vi "Telnet Parse AIC Command.vi"(11 "AIC sequence":string) -> (0 "error":bool, 1 "command":string, 2 "after sequence":string, 3 "AIC result":string, 4 "option negotiation":bool, 5 "sub option negotiation":bool, 6 "option info":T1)   [LabVIEW 2014]
panel:
  out "Recved /FF/FE":bool
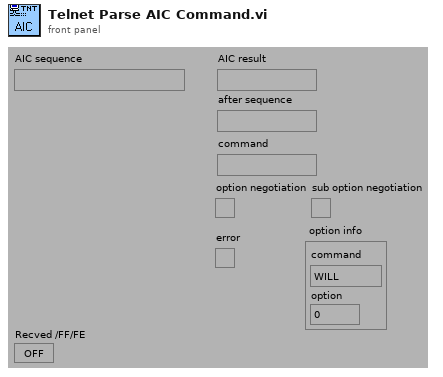
[diagram p1: front panel]
types:
  T1 = cluster{"command":enum16{"WILL", "WON'T", "DO", "DON'T"}, "option":u8}
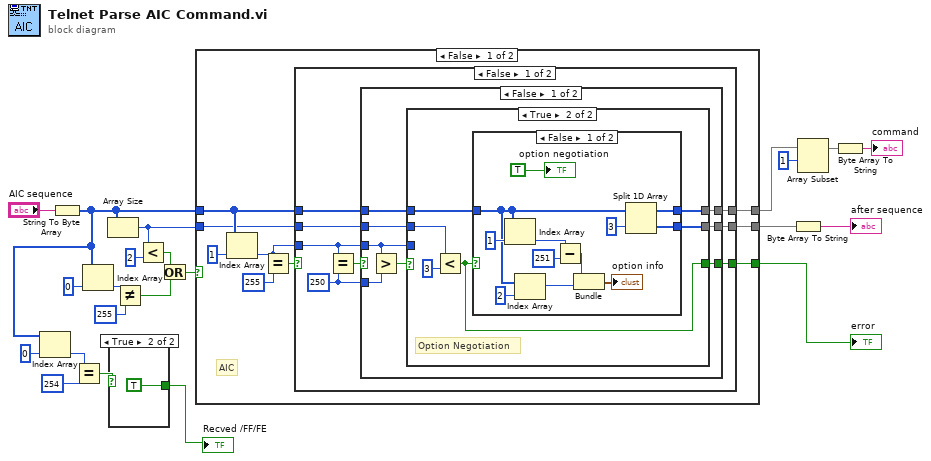
[diagram p0: block diagram]
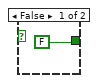
[diagram p2: hidden frame]
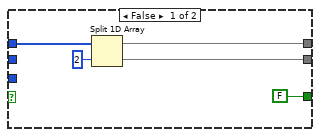
[diagram p3: hidden frame]
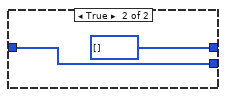
[diagram p4: hidden frame]
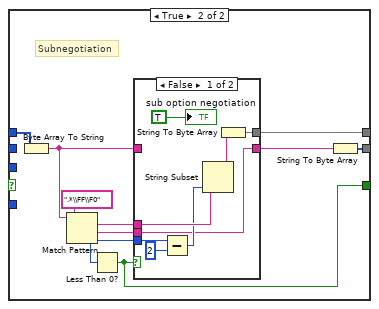
[diagram p5: hidden frame]
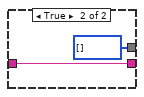
[diagram p6: hidden frame]
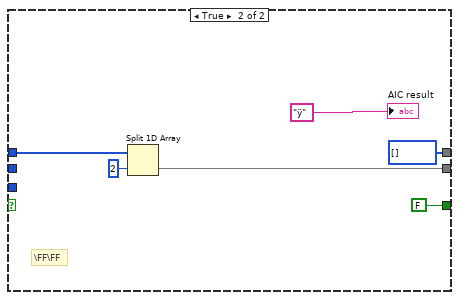
[diagram p7: hidden frame]
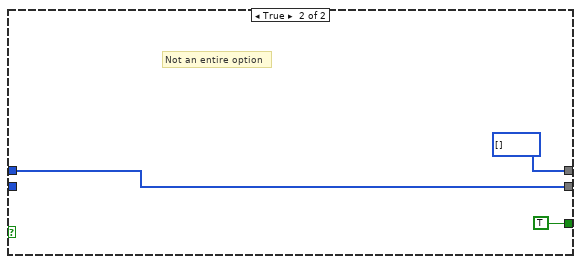
[diagram p8: hidden frame]
diagram:
  n1 = String To Byte Array(string="AIC sequence") -> (unsigned byte array=w5:u8[])
  n2 = Index Array(array=w5, index=0) -> (element=w4:u8)
  n3 = Equal?(x=w4, y=u8 254 ("x")) -> (x = y?=w2:bool)
  n4 = Index Array(array=w5, index=0) -> (element=w19:u8)
  n5 = Array Size(array=w5) -> (size(s)=w11:i32)
  n6 = case shown="True" w2 {
    tunnel: [FALSE TRUE] -> w1
    frame False {
    }
    frame True {
    }
  }
  "Recved /FF/FE" <- w1
  n7 = Not Equal?(x=w19, y=u8 255 ("x")) -> (x != y?=w18:bool)
  n8 = Less?(x=w11, y=2) -> (x < y?=w12:bool)
  n9 = Or(x=w12, y=w18) -> (x .or. y?=w13:bool)
  n10 = case shown="False" w13 {
    tunnel: w5 -> [w29 w102]
    tunnel: [w28 w102] -> w17
    tunnel: w11 -> [w27 _]
    tunnel: [w26 u8[] [] ("unsigned byte array")] -> w9
    tunnel: [w25 TRUE] -> w14
    frame False {
      # "AIC"
      n11 = Index Array(array=w29, index=1) -> (element=w31:u8)
      n12 = Equal?(x=w31, y=u8 255 ("x")) -> (x = y?=w30:bool)
      n13 = case shown="False" w30 {
        tunnel: w31 -> [w40 _]
        tunnel: w29 -> [w38 w100]
        tunnel: [w37 w98] -> w28
        tunnel: w27 -> [w36 _]
        tunnel: [w35 u8[] []] -> w26
        tunnel: [w34 FALSE] -> w25
        frame False {
          w41 = u8 250 ("x")
          n14 = Equal?(x=w40, y=w41) -> (x = y?=w39:bool)
          n15 = case shown="False" w39 {
            tunnel: w40 -> [w45 _]
            tunnel: w41 -> [w49 _]
            tunnel: w38 -> [w47 w84]
            tunnel: [w46 w82] -> w37
            tunnel: w36 -> [w44 _]
            tunnel: [w43 w76] -> w35
            tunnel: [w42 w75] -> w34
            frame False {
              n16 = Greater?(x=w45, y=w49) -> (0:w48:bool)
              n17 = case shown="True" w48 {
                tunnel: w47 -> [w54 w58]
                tunnel: [w52 w57] -> w46
                tunnel: w45 -> [_ _]
                tunnel: w44 -> [_ w59]
                tunnel: [w50 w56] -> w43
                tunnel: [FALSE w55] -> w42
                frame False {
                  n18 = Split 1D Array(array=w54, index=2) -> (first subarray=w50:u8[], second subarray=w52:u8[])
                }
                frame True {
                  # "Option Negotiation"
                  n19 = Less?(x=w59, y=3) -> (x < y?=w55:bool)
                  n20 = case shown="False" w55 {
                    tunnel: w58 -> [w62 w74]
                    tunnel: [w71 w74] -> w57
                    tunnel: [w70 u8[] []] -> w56
                    frame False {
                      n21 = Index Array(array=w62, index=1) -> (element=w67:u8)
                      n22 = Index Array(array=w62, index=2) -> (element=w61:u8)
                      n23 = Subtract(x=w67, y=u8 251) -> (x-y=w64:u8)
                      n24 = Bundle(w64, w61) -> (→"option info":cluster{u8, u8})  [unwired: 1 in]
                      n25 = Split 1D Array(array=w62, index=3) -> (first subarray=w70:u8[], second subarray=w71:u8[])
                      "option negotiation" <- TRUE ("option negotiation")
                    }
                    frame True {
                    }
                  }
                }
              }
            }
            frame True {
              # "Subnegotiation"
              n26 = Byte Array To String(unsigned byte array=w84) -> (string=w78:string)
              n27 = Match Pattern(string=w78, regular expression=".*\\FF\\F0") -> (match substring=w80:string, after substring=w77:string, offset past match=w81:i32)  [unwired: 1 in, 1 out]
              n28 = Less Than 0?(x=w81) -> (x < 0?=w75:bool)
              n29 = case shown="False" w75 {
                tunnel: w80 -> [w92 _]
                tunnel: w81 -> [w91 _]
                tunnel: [w88 w94] -> w79
                tunnel: w78 -> [_ w94]
                tunnel: w77 -> [w88 _]
                tunnel: [w86 u8[] [] ("unsigned byte array")] -> w76
                frame False {
                  n30 = Subtract(x=w91, y=2) -> (x-y=w89:i32)
                  n31 = String Subset(string=w92, length (rest)=w89) -> (substring=w87:string)  [unwired: 1 in]
                  n32 = String To Byte Array(string=w87) -> (unsigned byte array=w86:u8[])
                  "sub option negotiation" <- TRUE ("sub option negotiation")
                }
                frame True {
                }
              }
              n33 = String To Byte Array(string=w79) -> (unsigned byte array=w82:u8[])
            }
          }
        }
        frame True {
          # "\\FF\\FF"
          n34 = Split 1D Array(array=w100, index=2) -> (second subarray=w98:u8[])  [unwired: 1 out]
          "AIC result" <- "ÿ" ("AIC result")
        }
      }
    }
    frame True {
      # "Not an entire option"
    }
  }
  "error" <- w14
  n35 = Byte Array To String(unsigned byte array=w17) -> (string=→"after sequence":string)
  n36 = Array Subset(array=w9, index=1) -> (w7:u8[])  [unwired: 1 in]
  n37 = Byte Array To String(unsigned byte array=w7) -> (string=→"command":string)
